vi "Set Table Row Alarm.vi"(0 "Value":string[][](array[string]), 1 "Current Step ID":i32, 2 "Test Table":refnum<vi>) -> ()   [LabVIEW 2010]
uses:
  <vilib>/Utility/miscctls.llb/LVRowAndColumnTypeDef.ctl
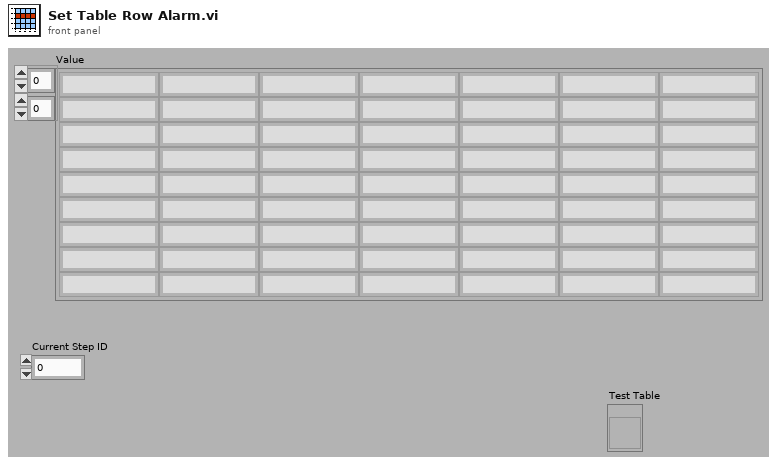
[diagram p1: front panel]
types:
  T1 = typedef "LVRowAndColumnTypeDef.ctl" = cluster{"Row":i32, "Column":i32}
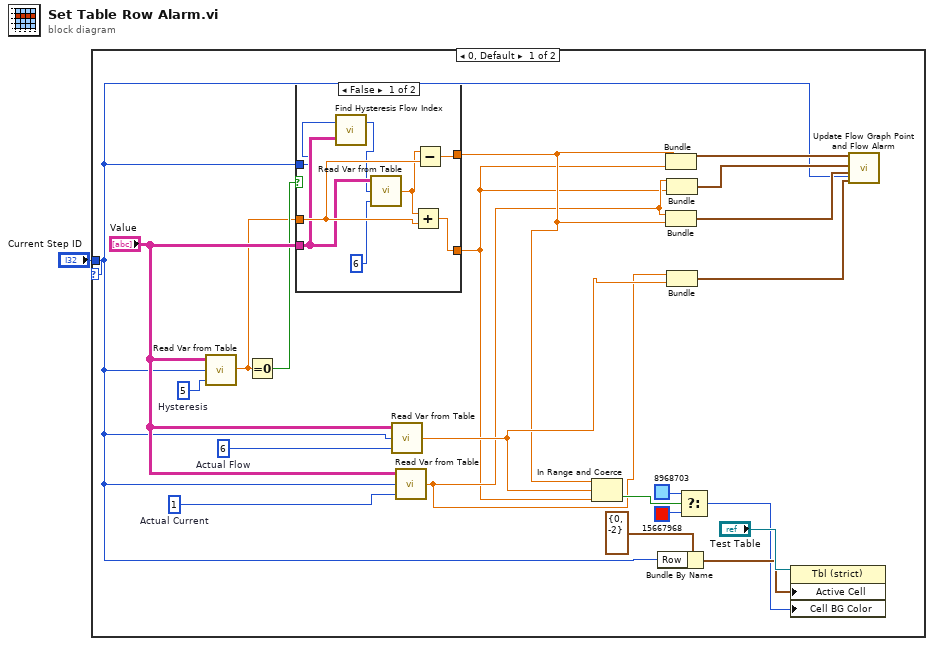
[diagram p0: block diagram]
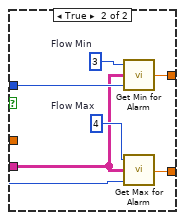
[diagram p2: hidden frame]
diagram:
  n1 = case shown="0, Default" "Current Step ID" {
    tunnel: "Current Step ID" -> [w5 _]
    frame 0, Default {
      w4 = 5  # Hysteresis
      w14 = 6  # Actual Flow
      w15 = 1  # Actual Current
      n2 = call "Read Var from Table.vi"("VAR Column Index"=w4, "Current Step ID"=w5, "Value"="Value") -> ("Numeric"=w2:dbl)
      n3 = Equal To 0?(x=w2) -> (x = 0?=w3:bool)
      n4 = case shown="False" w3 {
        tunnel: w5 -> [w25 w35]
        tunnel: "Value" -> [w26 w34]
        tunnel: [w31 w33] -> w9
        tunnel: [w30 w32] -> w7
        tunnel: w2 -> [w29 _]
        frame False {
          n5 = call "Find Hysteresis Flow Index.vi"("Value"=w26, "Current Step ID"=w25) -> ("Hysteresis Step ID"=w24:i32)  [unwired: 1 in]
          n6 = call "Read Var from Table.vi"("VAR Column Index"=6, "Current Step ID"=w24, "Value"=w26) -> ("Numeric"=w28:dbl)
          n7 = Add(x=w28, y=w29) -> (x+y=w30:dbl)
          n8 = Subtract(x=w28, y=w29) -> (x-y=w31:dbl)
        }
        frame True {
          w36 = 4  # Flow Max
          w37 = 3  # Flow Min
          n9 = call "Get Min for Alarm.vi"("Current Step Index"=w35, "Test Table"=w34, "Column Index for Min"=w37) -> ("Min"=w33:dbl)
          n10 = call "Get Max for Alarm.vi"("Current Step Index"=w35, "Test Table"=w34, "Column Index for Max"=w36) -> ("Min"=w32:dbl)
        }
      }
      n11 = call "Read Var from Table.vi"("VAR Column Index"=w14, "Current Step ID"=w5, "Value"="Value") -> ("Numeric"=w10:dbl)
      n12 = call "Read Var from Table.vi"("VAR Column Index"=w15, "Current Step ID"=w5, "Value"="Value") -> ("Numeric"=w8:dbl)
      n13 = In Range and Coerce(upper limit=w9, x=w10, lower limit=w7) -> (In Range?=w20:bool)  [unwired: 1 out]
      n14 = Bundle By Name(cluster=T1 {"Row"=0, "Column"=-2} ("Active Cell:Active Cell"), "Row"=w5) -> (w21:T1)
      n15 = Bundle("Min"=w9, "Min"=w7) -> (w16:cluster{"Min":dbl, "Min":dbl})  [unwired: 1 in]
      n16 = Bundle("Numeric"=w8, "Min"=w9) -> (w13:cluster{"Numeric":dbl, "Min":dbl})  [unwired: 1 in]
      n17 = Bundle("Numeric"=w8, "Min"=w7) -> (w12:cluster{"Numeric":dbl, "Min":dbl})  [unwired: 1 in]
      n18 = Bundle("Numeric"=w8, "Numeric"=w10) -> (w11:cluster{"Numeric":dbl, "Numeric":dbl})  [unwired: 1 in]
      n19 = Select(t=u32 8968703 ("Color Box"), s=w20, f=u32 15667968 ("Color Box")) -> (s? t:f=w17:u32)
      n20 = property class="Tbl (strict)"(reference="Test Table", "Active Cell"=w21, "Cell BG Color"=w17) -> ()  [unwired: 1 in, 2 out]
      n21 = call "Update Flow Graph Point and Flow Alarm.vi"("Current Step ID"=w5, "Actual Flow vs Current"=w11, "Low Flow Limit vs Current"=w13, "High Flow Limit vs Current"=w12, "Max and Min Flow"=w16) -> ()  [unwired: 2 in]
    }
    frame -1 {
    }
  }
